vi "Allocate Image Memory (Pattern).vi"() -> (0 "error out":errorcluster, 1 "Template":T1, 2 "Process Memory":T1, 3 "Acquisition Memory":T1[](array[typedef]))   [LabVIEW 2018]
uses:
  <vilib>/vision/Image Controls.llb/IMAQ Image.ctl
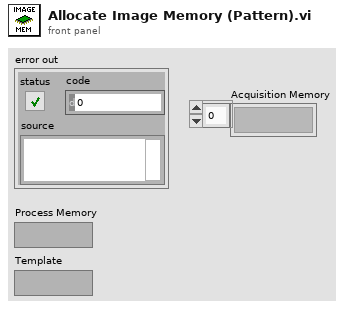
[diagram p1: front panel]
types:
  T1 = typedef "IMAQ Image.ctl" = refnum<image>
  T2 = typedef "Image Type" = u32
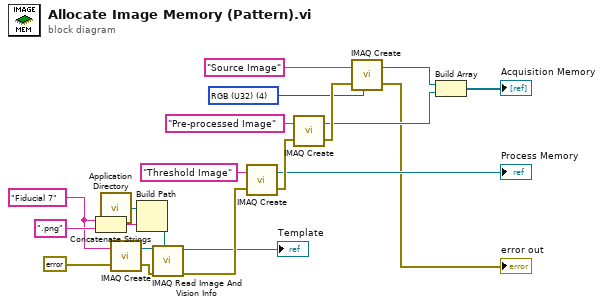
[diagram p0: block diagram]
diagram:
  w2 = "Fiducial 7"
  w12 = T2 4 items=["Grayscale (U8)", "Grayscale (I16)", "Grayscale (SGL)", "Complex (CSG)", "RGB (U32)", "HSL (U32)", "RGB (U64)", "Grayscale (U16)"] ("Image Type")
  n1 = Concatenate Strings(w2, ".png" ("string")) -> (w5:string)
  n2 = call <vilib>:"Application Directory.vi"() -> ("Application Directory"=w6:path)
  n3 = call "IMAQ Create"("Image Name"=w2, "error in (no error)"=errorcluster {"status"=FALSE, "code"=0, "source"=""} ("error out")) -> ("New Image"=w8:T1, "error out"=w3:errorcluster)  [unwired: 3 in]
  n4 = Build Path(base path=w6, name or relative path=w5) -> (appended path=w7:path)
  n5 = call "IMAQ Read Image And Vision Info"("File Path"=w7, "error in (no error)"=w3, "Image"=w8) -> ("error out"=w10:errorcluster, "Image Out"=→"Template":T1)  [unwired: 6 in, 1 out]
  n6 = call "IMAQ Create"("Image Name"="Threshold Image", "error in (no error)"=w10) -> ("New Image"=→"Process Memory":T1, "error out"=w19:errorcluster)  [unwired: 3 in]
  n7 = call "IMAQ Create"("Image Name"="Pre-processed Image", "error in (no error)"=w19) -> ("New Image"=w15:T1, "error out"=w16:errorcluster)  [unwired: 3 in]
  n8 = call "IMAQ Create"("Image Name"="Source Image", "Image Type"=w12, "error in (no error)"=w16) -> ("New Image"=w14:T1, "error out"=→"error out":errorcluster)  [unwired: 2 in]
  n9 = Build Array(w14, w15) -> (→"Acquisition Memory":T1[])
